vi "Check Paths.vi"(11 "Glue Pathways":T2 {"BBM Slot" items=["Slot 1", "Slot 2", "Slot 3", "Slot 4"]; "Weight Slot" items=["Slot 1", "Slot 2", "Slot 3", "Slot 4"]; "Glue Slot" items=["Slot 1", "Slot 2", "Slot 3", "Slot 4"]; "Stamp Slot" items=["Slot 1", "Slot 2", "Slot 3", "Slot 4"]; "HDI Slot" items=["Slot 1", "Slot 2", "Slot 3", "Slot 4"]}) -> (3 "Active Paths":T1)   [LabVIEW 2011]
uses:
  UI typedefs/Glue Paths.ctl
  UI typedefs/Glue Path.ctl
  UI typedefs/Active Paths.ctl
  UI typedefs/Weight Chuck Control.ctl
  UI typedefs/Weight Slot Control.ctl
  Shared Components/Config Manager Class/Type Definitions/Weight Type.ctl
  UI typedefs/Stamp Chuck Control.ctl
  UI typedefs/Stamp Slot Control.ctl
  Shared Components/Config Manager Class/Type Definitions/Stamp Type.ctl
  UI typedefs/HDI Chuck Control.ctl
  UI typedefs/HDI Slot Control.ctl
  UI typedefs/Glue Chuck Control.ctl
  UI typedefs/Glue Slot Control.ctl
  UI typedefs/BM Chuck Control.ctl
  UI typedefs/BM Slot Control.ctl
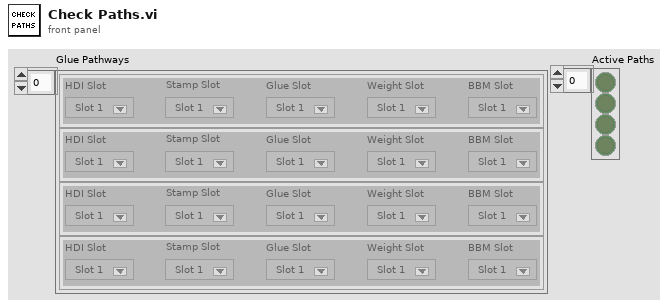
[diagram p1: front panel]
types:
  T1 = typedef "Active Paths.ctl" = bool[]
  T2 = typedef "Glue Paths.ctl" = T3[]
  T3 = typedef "Glue Path.ctl" = cluster{"HDI Slot ":i32, "Stamp Slot":u32, "Glue Slot":i32, "Weight Slot":i32, "BBM Slot":i32}
  T4 = typedef "Weight Chuck Control.ctl" = cluster{"Slot 1":T5, "Slot 2":T5, "Slot 3":T5, "Slot 4":T5}
  T5 = typedef "Weight Slot Control.ctl" = cluster{"Populated?":bool, "Weight Type":T6}
  T6 = typedef "Weight Type.ctl" = enum16{"Weight 1", "Weight 2", "Weight 3", "Weight 4", "Weight 5", "Weight 6", "Weight 7", "Weight 8"}
  T7 = typedef "Stamp Chuck Control.ctl" = cluster{"Slot 1":T8, "Slot 2":T8, "Slot 3":T8, "Slot 4":T8}
  T8 = typedef "Stamp Slot Control.ctl" = cluster{"Populated?":bool, "Stamp Type":T9}
  T9 = typedef "Stamp Type.ctl" = enum16{"Stamp 1", "Stamp 2", "Stamp 3", "Stamp 4", "Stamp 5"}
  T10 = typedef "HDI Chuck Control.ctl" = cluster{"Slot 1":T11, "Slot 2":T11, "Slot 3":T11, "Slot 4":T11}
  T11 = typedef "HDI Slot Control.ctl" = cluster{"Populated?":bool, "Identification:":string}
  T12 = typedef "Glue Chuck Control.ctl" = cluster{"Slot 1":T13, "Slot 2":T13, "Slot 3":T13, "Slot 4":T13}
  T13 = typedef "Glue Slot Control.ctl" = cluster{"Populated?":bool}
  T14 = typedef "BM Chuck Control.ctl" = cluster{"Slot 1":T15, "Slot 2":T15, "Slot 3":T15, "Slot 4":T15}
  T15 = typedef "BM Slot Control.ctl" = cluster{"Populated?":bool}
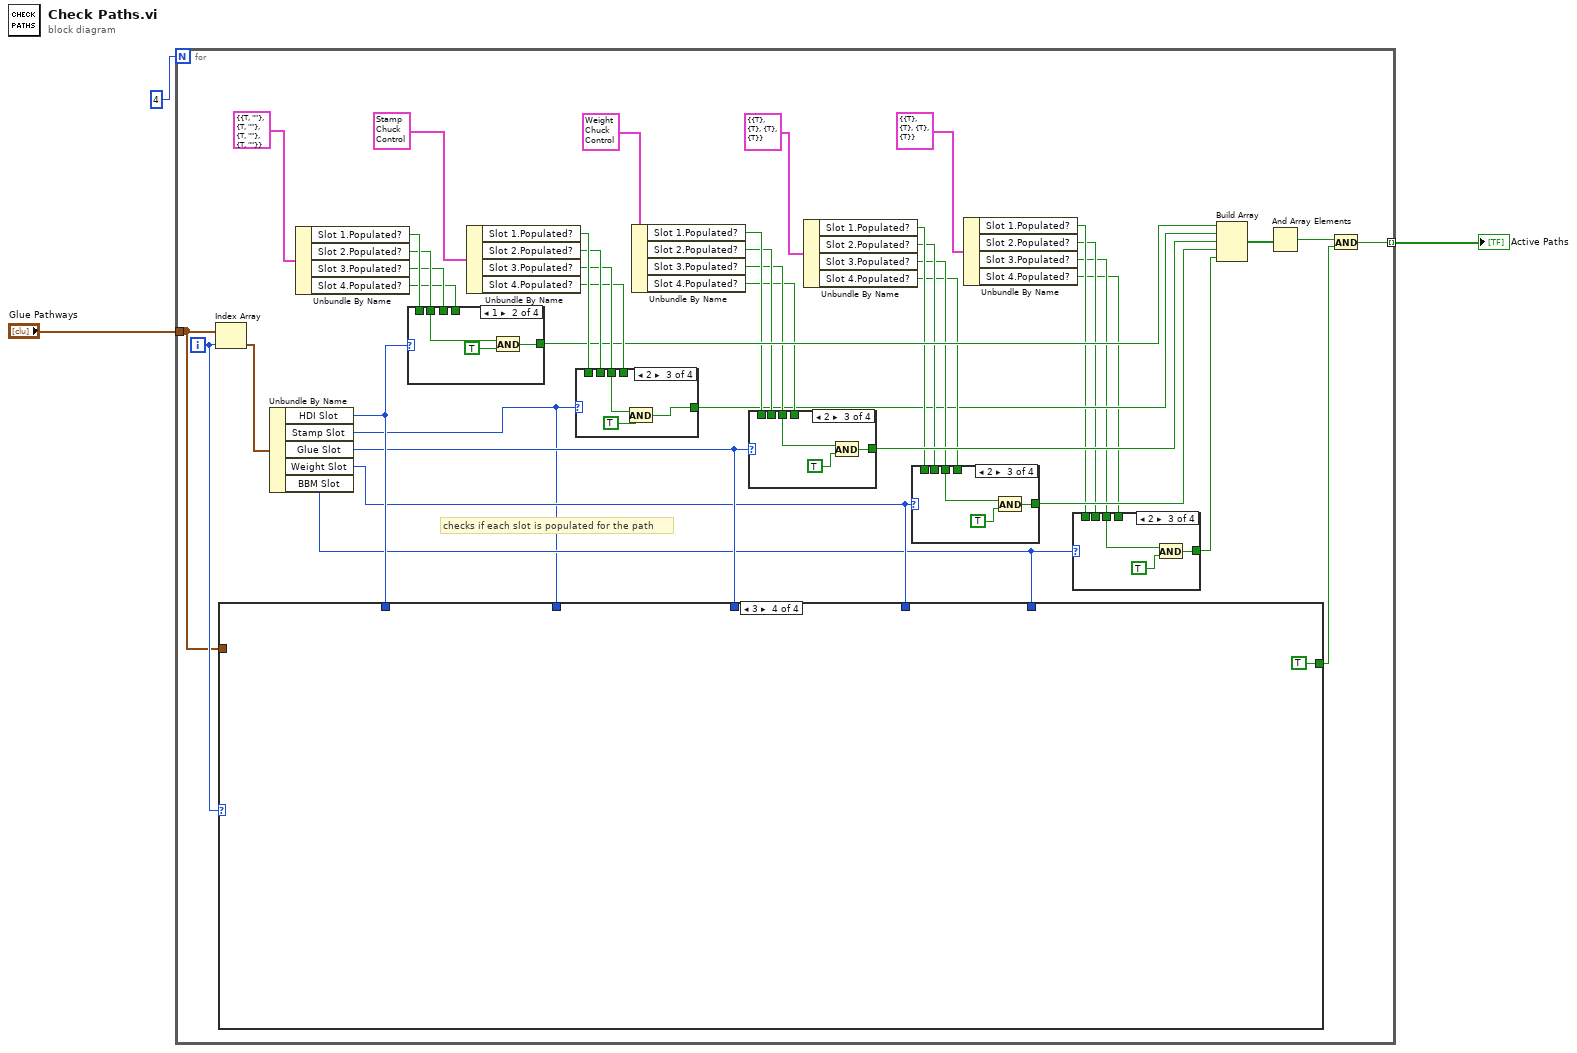
[diagram p0: block diagram]
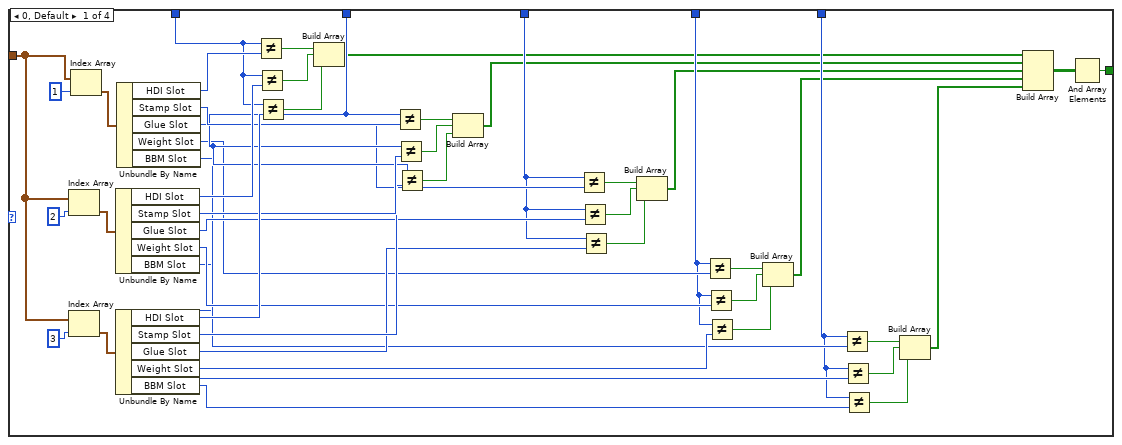
[diagram p2: hidden frame]
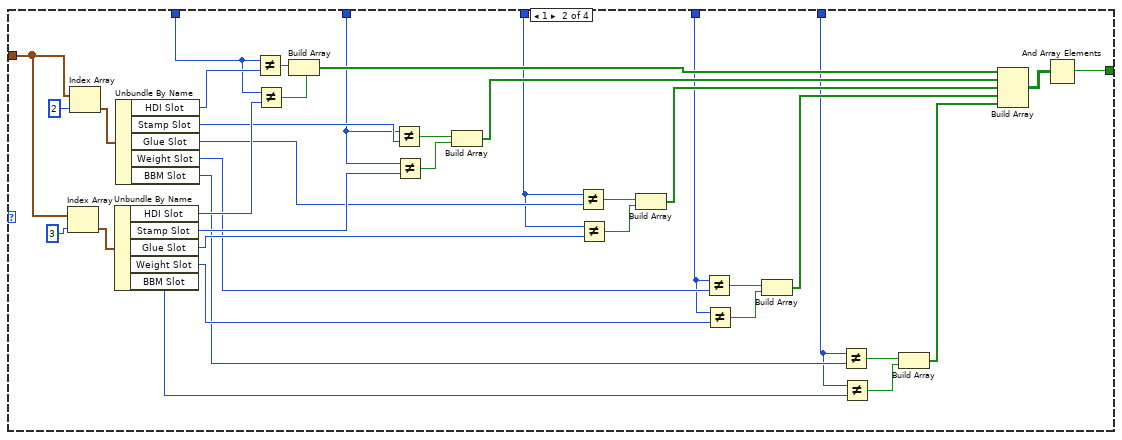
[diagram p3: hidden frame]
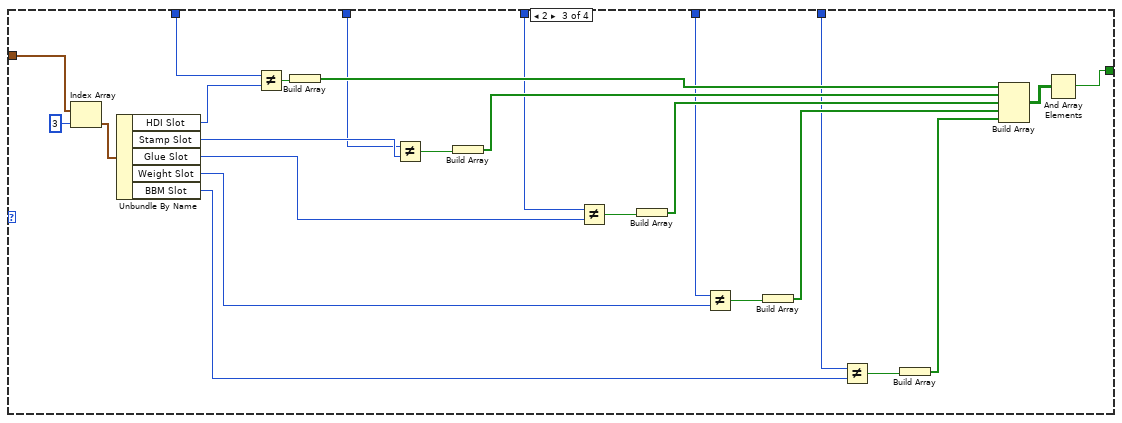
[diagram p4: hidden frame]
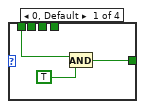
[diagram p5: hidden frame]
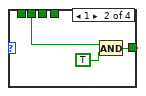
[diagram p6: hidden frame]
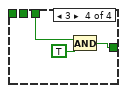
[diagram p7: hidden frame]
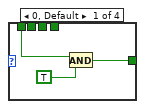
[diagram p8: hidden frame]
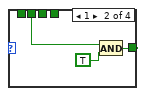
[diagram p9: hidden frame]
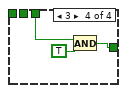
[diagram p10: hidden frame]
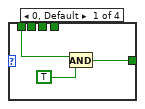
[diagram p11: hidden frame]
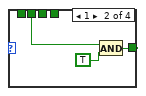
[diagram p12: hidden frame]
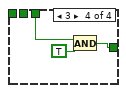
[diagram p13: hidden frame]
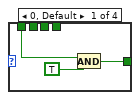
[diagram p14: hidden frame]
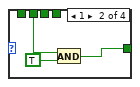
[diagram p15: hidden frame]
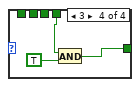
[diagram p16: hidden frame]
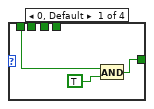
[diagram p17: hidden frame]
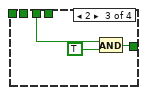
[diagram p18: hidden frame]
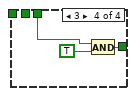
[diagram p19: hidden frame]
diagram:
  n1 = for {
    N: 4 -> [_]
    tunnel: "Glue Pathways" -> [w5]
    tunnel: [w7] -> w1 mode=indexing
    i -> [w6]
    # "checks if each slot is populated for the path"
    n2 = Index Array(array=w5, index=w6) -> (element=w13:T3)
    n3 = Unbundle By Name(w13) -> ("HDI Slot"=w19:i32, "Stamp Slot"=w4:u32, "Glue Slot"=w18:i32, "Weight Slot"=w17:i32, "BBM Slot"=w16:i32)
    n4 = case shown="3" w6 {
      tunnel: w19 -> [w86 w100 w137 _]
      tunnel: w4 -> [w69 w99 w136 _]
      tunnel: w18 -> [w66 w98 w135 _]
      tunnel: w17 -> [w62 w97 w134 _]
      tunnel: w16 -> [w55 w96 w133 _]
      tunnel: [w47 w102 w132 TRUE] -> w14
      tunnel: w5 -> [w46 w101 w138 _]
      frame 0, Default {
        n5 = Index Array(array=w46, index=2) -> (element=w90:T3)
        n6 = Index Array(array=w46, index=3) -> (element=w89:T3)
        n7 = Index Array(array=w46, index=1) -> (element=w91:T3)
        n8 = Unbundle By Name(w90) -> ("HDI Slot"=w87:i32, "Stamp Slot"=w71:u32, "Glue Slot"=w67:i32, "Weight Slot"=w63:i32, "BBM Slot"=w56:i32)
        n9 = Unbundle By Name(w89) -> ("HDI Slot"=w85:i32, "Stamp Slot"=w70:u32, "Glue Slot"=w65:i32, "Weight Slot"=w61:i32, "BBM Slot"=w54:i32)
        n10 = Unbundle By Name(w91) -> ("HDI Slot"=w88:i32, "Stamp Slot"=w72:u32, "Glue Slot"=w68:i32, "Weight Slot"=w64:i32, "BBM Slot"=w57:i32)
        n11 = Not Equal?(x=w86, y=w88) -> (x != y?=w84:bool)
        n12 = Not Equal?(x=w86, y=w87) -> (x != y?=w83:bool)
        n13 = Not Equal?(x=w86, y=w85) -> (x != y?=w82:bool)
        n14 = Build Array(w84, w83, w82) -> (w53:bool[])
        n15 = Not Equal?(x=w69, y=w72) -> (x != y?=w79:bool)
        n16 = Not Equal?(x=w69, y=w71) -> (x != y?=w80:bool)
        n17 = Not Equal?(x=w69, y=w70) -> (x != y?=w81:bool)
        n18 = Build Array(w79, w80, w81) -> (w52:bool[])
        n19 = Not Equal?(x=w66, y=w68) -> (x != y?=w73:bool)
        n20 = Not Equal?(x=w66, y=w67) -> (x != y?=w74:bool)
        n21 = Not Equal?(x=w66, y=w65) -> (x != y?=w75:bool)
        n22 = Build Array(w73, w74, w75) -> (w51:bool[])
        n23 = Not Equal?(x=w62, y=w64) -> (x != y?=w78:bool)
        n24 = Not Equal?(x=w62, y=w63) -> (x != y?=w77:bool)
        n25 = Not Equal?(x=w62, y=w61) -> (x != y?=w76:bool)
        n26 = Build Array(w78, w77, w76) -> (w50:bool[])
        n27 = Not Equal?(x=w55, y=w57) -> (x != y?=w58:bool)
        n28 = Not Equal?(x=w55, y=w56) -> (x != y?=w59:bool)
        n29 = Not Equal?(x=w55, y=w54) -> (x != y?=w60:bool)
        n30 = Build Array(w58, w59, w60) -> (w49:bool[])
        n31 = Build Array(w53, w52, w51, w50, w49) -> (w48:bool[][])
        n32 = And Array Elements(Boolean array=w48) -> (logical AND=w47:bool)
      }
      frame 1 {
        n33 = Index Array(array=w101, index=3) -> (element=w128:T3)
        n34 = Index Array(array=w101, index=2) -> (element=w129:T3)
        n35 = Unbundle By Name(w128) -> ("HDI Slot"=w126:i32, "Stamp Slot"=w116:u32, "Glue Slot"=w114:i32, "Weight Slot"=w112:i32, "BBM Slot"=w95:i32)
        n36 = Unbundle By Name(w129) -> ("HDI Slot"=w127:i32, "Stamp Slot"=w117:u32, "Glue Slot"=w115:i32, "Weight Slot"=w113:i32, "BBM Slot"=w109:i32)
        n37 = Not Equal?(x=w100, y=w127) -> (x != y?=w125:bool)
        n38 = Not Equal?(x=w100, y=w126) -> (x != y?=w124:bool)
        n39 = Build Array(w125, w124) -> (w108:bool[])
        n40 = Not Equal?(x=w99, y=w117) -> (x != y?=w122:bool)
        n41 = Not Equal?(x=w99, y=w116) -> (x != y?=w123:bool)
        n42 = Build Array(w122, w123) -> (w107:bool[])
        n43 = Not Equal?(x=w98, y=w115) -> (x != y?=w118:bool)
        n44 = Not Equal?(x=w98, y=w114) -> (x != y?=w119:bool)
        n45 = Build Array(w118, w119) -> (w106:bool[])
        n46 = Not Equal?(x=w97, y=w113) -> (x != y?=w121:bool)
        n47 = Not Equal?(x=w97, y=w112) -> (x != y?=w120:bool)
        n48 = Build Array(w121, w120) -> (w105:bool[])
        n49 = Not Equal?(x=w96, y=w109) -> (x != y?=w110:bool)
        n50 = Not Equal?(x=w96, y=w95) -> (x != y?=w111:bool)
        n51 = Build Array(w110, w111) -> (w104:bool[])
        n52 = Build Array(w108, w107, w106, w105, w104) -> (w103:bool[][])
        n53 = And Array Elements(Boolean array=w103) -> (logical AND=w102:bool)
      }
      frame 2 {
        n54 = Index Array(array=w138, index=3) -> (element=w155:T3)
        n55 = Unbundle By Name(w155) -> ("HDI Slot"=w154:i32, "Stamp Slot"=w149:u32, "Glue Slot"=w148:i32, "Weight Slot"=w147:i32, "BBM Slot"=w145:i32)
        n56 = Not Equal?(x=w137, y=w154) -> (x != y?=w153:bool)
        n57 = Build Array(w153) -> (w144:bool[])
        n58 = Not Equal?(x=w136, y=w149) -> (x != y?=w152:bool)
        n59 = Build Array(w152) -> (w143:bool[])
        n60 = Not Equal?(x=w135, y=w148) -> (x != y?=w150:bool)
        n61 = Build Array(w150) -> (w142:bool[])
        n62 = Not Equal?(x=w134, y=w147) -> (x != y?=w151:bool)
        n63 = Build Array(w151) -> (w141:bool[])
        n64 = Not Equal?(x=w133, y=w145) -> (x != y?=w146:bool)
        n65 = Build Array(w146) -> (w140:bool[])
        n66 = Build Array(w144, w143, w142, w141, w140) -> (w139:bool[][])
        n67 = And Array Elements(Boolean array=w139) -> (logical AND=w132:bool)
      }
      frame 3 {
      }
    }
    n68 = Unbundle By Name(T10 {"Slot 1"={"Populated?"=TRUE, "Identification:"=""}, "Slot 2"={"Populated?"=TRUE, "Identification:"=""}, "Slot 3"={"Populated?"=TRUE, "Identification:"=""}, "Slot 4"={"Populated?"=TRUE, "Identification:"=""}} ("HDI Chuck Control")) -> ("Slot 1.Populated?"=w45:bool, "Slot 2.Populated?"=w44:bool, "Slot 3.Populated?"=w43:bool, "Slot 4.Populated?"=w42:bool)
    n69 = case shown="1" w19 {
      tunnel: w45 -> [w207 _ _ _]
      tunnel: [w206 w209 w212 w216] -> w37
      tunnel: w44 -> [_ w211 _ _]
      tunnel: w43 -> [_ _ w214 _]
      tunnel: w42 -> [_ _ _ w215]
      frame 0, Default {
        n70 = And(x=w207, y=TRUE) -> (x .and. y?=w206:bool)
      }
      frame 1 {
        n71 = And(x=w211, y=TRUE) -> (x .and. y?=w209:bool)
      }
      frame 2 {
        n72 = And(x=w214, y=TRUE) -> (x .and. y?=w212:bool)
      }
      frame 3 {
        n73 = And(x=w215, y=TRUE) -> (x .and. y?=w216:bool)
      }
    }
    n74 = Unbundle By Name(T7 {"Slot 1"={"Populated?"=TRUE, "Stamp Type"=enum."Stamp 1"}, "Slot 2"={"Populated?"=TRUE, "Stamp Type"=enum."Stamp 2"}, "Slot 3"={"Populated?"=TRUE, "Stamp Type"=enum."Stamp 3"}, "Slot 4"={"Populated?"=TRUE, "Stamp Type"=enum."Stamp 4"}} ("Stamp Chuck Control")) -> ("Slot 1.Populated?"=w41:bool, "Slot 2.Populated?"=w40:bool, "Slot 3.Populated?"=w39:bool, "Slot 4.Populated?"=w38:bool)
    n75 = case shown="2" w4 {
      tunnel: [w195 w198 w200 w204] -> w24
      tunnel: w41 -> [w194 _ _ _]
      tunnel: w39 -> [_ _ w202 _]
      tunnel: w40 -> [_ w197 _ _]
      tunnel: w38 -> [_ _ _ w203]
      frame 0, Default {
        n76 = And(x=w194, y=TRUE) -> (x .and. y?=w195:bool)
      }
      frame 1 {
        n77 = And(x=w197, y=TRUE) -> (x .and. y?=w198:bool)
      }
      frame 2 {
        n78 = And(x=w202, y=TRUE) -> (x .and. y?=w200:bool)
      }
      frame 3 {
        n79 = And(x=w203, y=TRUE) -> (x .and. y?=w204:bool)
      }
    }
    n80 = Unbundle By Name(T4 {"Slot 1"={"Populated?"=TRUE, "Weight Type"=enum."Weight 1"}, "Slot 2"={"Populated?"=TRUE, "Weight Type"=enum."Weight 2"}, "Slot 3"={"Populated?"=TRUE, "Weight Type"=enum."Weight 3"}, "Slot 4"={"Populated?"=TRUE, "Weight Type"=enum."Weight 4"}} ("Weight Chuck Control")) -> ("Slot 1.Populated?"=w34:bool, "Slot 2.Populated?"=w33:bool, "Slot 3.Populated?"=w32:bool, "Slot 4.Populated?"=w31:bool)
    n81 = case shown="2" w18 {
      tunnel: [w183 w186 w189 w192] -> w35
      tunnel: w34 -> [w182 _ _ _]
      tunnel: w33 -> [_ w185 _ _]
      tunnel: w32 -> [_ _ w188 _]
      tunnel: w31 -> [_ _ _ w191]
      frame 0, Default {
        n82 = And(x=w182, y=TRUE) -> (x .and. y?=w183:bool)
      }
      frame 1 {
        n83 = And(x=w185, y=TRUE) -> (x .and. y?=w186:bool)
      }
      frame 2 {
        n84 = And(x=w188, y=TRUE) -> (x .and. y?=w189:bool)
      }
      frame 3 {
        n85 = And(x=w191, y=TRUE) -> (x .and. y?=w192:bool)
      }
    }
    n86 = Unbundle By Name(T12 {"Slot 1"={"Populated?"=TRUE}, "Slot 2"={"Populated?"=TRUE}, "Slot 3"={"Populated?"=TRUE}, "Slot 4"={"Populated?"=TRUE}} ("Glue Chuck Control")) -> ("Slot 1.Populated?"=w30:bool, "Slot 2.Populated?"=w29:bool, "Slot 3.Populated?"=w28:bool, "Slot 4.Populated?"=w27:bool)
    n87 = case shown="2" w17 {
      tunnel: [w171 w174 w177 w180] -> w26
      tunnel: w30 -> [w170 _ _ _]
      tunnel: w29 -> [_ w173 _ _]
      tunnel: w28 -> [_ _ w176 _]
      tunnel: w27 -> [_ _ _ w179]
      frame 0, Default {
        n88 = And(x=w170, y=TRUE) -> (x .and. y?=w171:bool)
      }
      frame 1 {
        n89 = And(x=w173, y=TRUE) -> (x .and. y?=w174:bool)
      }
      frame 2 {
        n90 = And(x=w176, y=TRUE) -> (x .and. y?=w177:bool)
      }
      frame 3 {
        n91 = And(x=w179, y=TRUE) -> (x .and. y?=w180:bool)
      }
    }
    n92 = Unbundle By Name(T14 {"Slot 1"={"Populated?"=TRUE}, "Slot 2"={"Populated?"=TRUE}, "Slot 3"={"Populated?"=TRUE}, "Slot 4"={"Populated?"=TRUE}} ("BM Chuck Control")) -> ("Slot 1.Populated?"=w23:bool, "Slot 2.Populated?"=w22:bool, "Slot 3.Populated?"=w21:bool, "Slot 4.Populated?"=w20:bool)
    n93 = case shown="2" w16 {
      tunnel: [w159 w162 w165 w168] -> w25
      tunnel: w23 -> [w158 _ _ _]
      tunnel: w22 -> [_ w161 _ _]
      tunnel: w21 -> [_ _ w164 _]
      tunnel: w20 -> [_ _ _ w167]
      frame 0, Default {
        n94 = And(x=w158, y=TRUE) -> (x .and. y?=w159:bool)
      }
      frame 1 {
        n95 = And(x=w161, y=TRUE) -> (x .and. y?=w162:bool)
      }
      frame 2 {
        n96 = And(x=w164, y=TRUE) -> (x .and. y?=w165:bool)
      }
      frame 3 {
        n97 = And(x=w167, y=TRUE) -> (x .and. y?=w168:bool)
      }
    }
    n98 = Build Array(w37, w24, w35, w26, w25) -> (w36:bool[])
    n99 = And Array Elements(Boolean array=w36) -> (logical AND=w15:bool)
    n100 = And(x=w15, y=w14) -> (x .and. y?=w7:bool)
  }
  "Active Paths" <- w1
